vi "ExDebugClose.vi"() -> ()   [LabVIEW 2010]
uses:
  GlobalSpectHdl.vi
  GlobalCamOpen.vi
  GlobalCamHandle.vi
panel:
  out "error out":errorcluster
  in  "error in (no error)":errorcluster
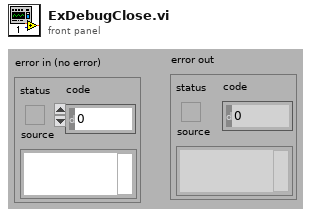
[diagram p1: front panel]
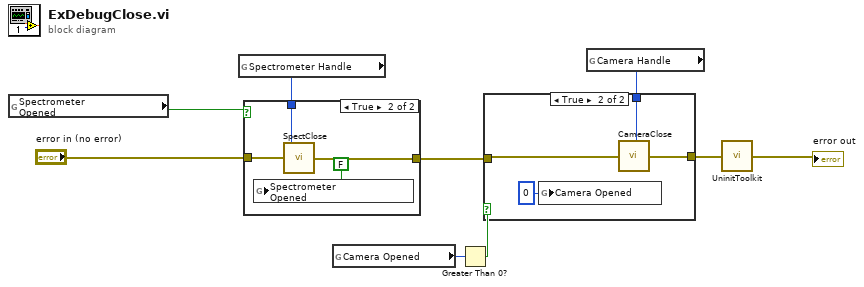
[diagram p0: block diagram]
diagram:
  n1 = global read "GlobalSpectHdl.vi" "Spectrometer \nOpened"() -> (w7:bool)
  n2 = global read "GlobalSpectHdl.vi" "Spectrometer Handle"() -> (w5:u32)
  n3 = case shown="True" w7 {
    tunnel: "error in (no error)" -> [w10 w14]
    tunnel: [w10 w13] -> w4
    tunnel: w5 -> [_ w12]
    frame False {
    }
    frame True {
      n4 = global write "GlobalSpectHdl.vi" "Spectrometer \nOpened"(FALSE) -> ()
      n5 = call <userlib>:"SpectClose.vi"("error in"=w14, "Spectrometer Handle"=w12) -> ("error out"=w13:errorcluster)
    }
  }
  n6 = global read "GlobalCamOpen.vi" "Camera Opened"() -> (w9:u32)
  n7 = Greater Than 0?(x=w9) -> (x > 0?=w8:bool)
  n8 = global read "GlobalCamHandle.vi" "Camera Handle"() -> (w3:u32)
  n9 = case shown="True" w8 {
    tunnel: w4 -> [w15 w19]
    tunnel: [w15 w18] -> w2
    tunnel: w3 -> [_ w17]
    frame False {
    }
    frame True {
      n10 = global write "GlobalCamOpen.vi" "Camera Opened"(0) -> ()
      n11 = call <userlib>:"CameraClose.vi"("error in"=w19, "Camera Handle"=w17) -> ("error out"=w18:errorcluster)
    }
  }
  n12 = call <userlib>:"UninitToolkit.vi"("error in"=w2) -> ("error out"=→"error out":errorcluster)
